vi "GetText.vi"(8 "error in":errorcluster, 11 "BuckBoost editor node in":refnum<class "BuckBoost editor node.lvclass">) -> (0 "error out":errorcluster, 1 "additional text":string, 2 "text":string, 3 "BuckBoost editor node out":refnum<class "BuckBoost editor node.lvclass">, 4 "glyph":string)   [LabVIEW 2017, in "BuckBoost editor node.lvclass"]
uses:
  BuckBoost editor node.lvclass
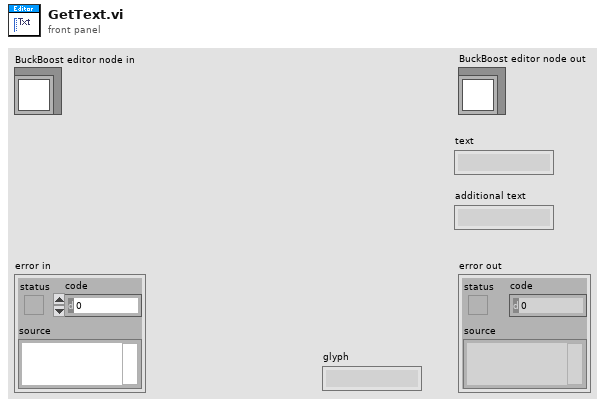
[diagram p1: front panel]
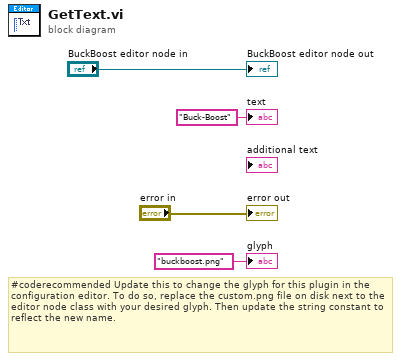
[diagram p0: block diagram]
diagram:
  # "#coderecommended Update this to change the glyph for this plugin in the configuration editor. To do so, replace the custom.png file on disk next to the editor node class with your desired glyph. Then update the string constant to reflect the new name."
  "error out" <- "error in"
  "BuckBoost editor node out" <- "BuckBoost editor node in"
  "text" <- "Buck-Boost" ("text")
  "glyph" <- "buckboost.png" ("glyph")
